vi "JSONHack.vi"(9 "search name":string, 11 "JSON in":string) -> (0 "Property (time stamp)":timestamp, 1 "Property (num)":dbl, 2 "Property (str)":string, 3 "What is left":string)   [LabVIEW 2019]
uses:
  <vilib>/Utility/miscctls.llb/LVDateTimeRec.ctl
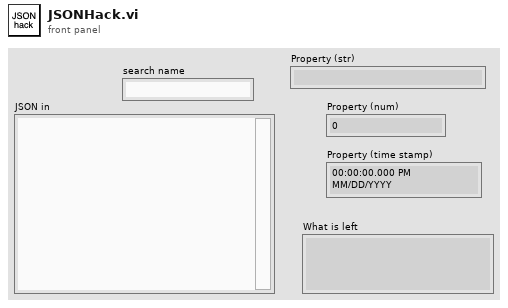
[diagram p1: front panel]
types:
  T1 = typedef "LVDateTimeRec.ctl" = cluster{"fractional second":dbl, "second":i32, "minute":i32, "hour":i32, "day of month":i32, "month":i32, "year":i32, "day of week":i32, "day of year":i32, "DST":i32}
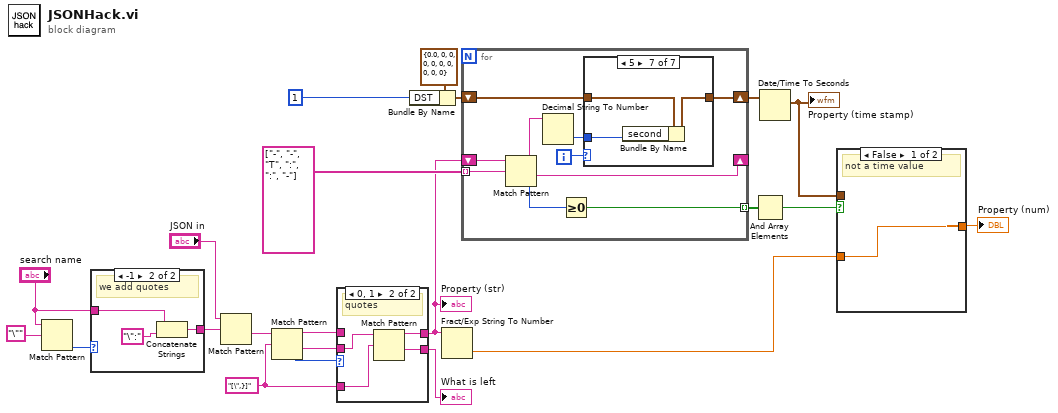
[diagram p0: block diagram]
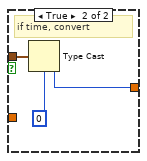
[diagram p2: hidden frame]
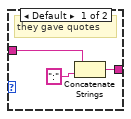
[diagram p4: hidden frame]
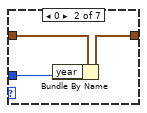
[diagram p6: hidden frame]
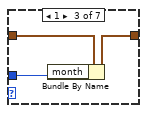
[diagram p7: hidden frame]
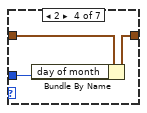
[diagram p8: hidden frame]
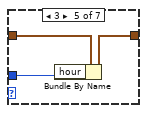
[diagram p9: hidden frame]
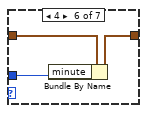
[diagram p10: hidden frame]
diagram:
  w9 = "[\",}]" ("regular expression")
  n1 = Match Pattern(string="search name", regular expression="\"" ("string")) -> (offset past match=w13:i32)  [unwired: 1 in, 3 out]
  n2 = case shown="-1" w13 {
    tunnel: [w24 w27] -> w20
    tunnel: "search name" -> [w23 w26]
    frame Default {
      # "they gave quotes"
      n3 = Concatenate Strings(w23, ":" ("string")) -> (w24:string)
    }
    frame -1 {
      # "we add quotes"
      n4 = Concatenate Strings(w26, "\":" ("string")) -> (w27:string)
    }
  }
  n5 = Match Pattern(string="JSON in", regular expression=w20) -> (after substring=w22:string)  [unwired: 1 in, 3 out]
  n6 = Match Pattern(string=w22, regular expression=w9) -> (before substring=w6:string, after substring=w10:string, offset past match=w11:i32)  [unwired: 1 in, 1 out]
  n7 = case shown="0, 1" w11 {
    tunnel: w10 -> [w30 w34]
    tunnel: w9 -> [_ w33]
    tunnel: [w30 w32] -> w8
    tunnel: [w29 w31] -> w7
    tunnel: w6 -> [w29 _]
    frame Default {
      # "number"
    }
    frame 0, 1 {
      # "quotes"
      n8 = Match Pattern(string=w34, regular expression=w33) -> (before substring=w31:string, after substring=w32:string)  [unwired: 1 in, 2 out]
    }
  }
  "Property (str)" <- w7
  "What is left" <- w8
  n9 = Bundle By Name(cluster=T1 {"fractional second"=0.0, "second"=0, "minute"=0, "hour"=0, "day of month"=0, "month"=0, "year"=0, "day of week"=0, "day of year"=0, "DST"=0} ("date time rec"), "DST"=1) -> (w15:T1)
  n10 = Fract/Exp String To Number(string=w7) -> (number=w3:dbl)  [unwired: 3 in, 1 out]
  n11 = for {
    tunnel: string[] ["-", "-", "T", ":", ":", "-"] -> [w43] mode=indexing
    shift-right: [w41] -> _
    shift-left: w7 -> [w44]
    shift-right: [w40] -> w18
    shift-left: w15 -> [w37]
    tunnel: [w35] -> w5 mode=indexing
    i -> [w39]
    n12 = Match Pattern(string=w44, regular expression=w43) -> (before substring=w42:string, after substring=w41:string, offset past match=w36:i32)  [unwired: 1 in, 1 out]
    n13 = Decimal String To Number(string=w42) -> (number=w38:i32)  [unwired: 2 in, 1 out]
    n14 = Greater Or Equal To 0?(x=w36) -> (x >= 0?=w35:bool)
    n15 = case shown="5" w39 {
      tunnel: w37 -> [w45 w48 w51 w54 w57 w60 w63]
      tunnel: [w45 w47 w50 w53 w56 w59 w62] -> w40
      tunnel: w38 -> [_ w46 w49 w52 w55 w58 w61]
      frame Default {
      }
      frame 0 {
        n16 = Bundle By Name(cluster=w48, "year"=w46) -> (w47:T1)
      }
      frame 1 {
        n17 = Bundle By Name(cluster=w51, "month"=w49) -> (w50:T1)
      }
      frame 2 {
        n18 = Bundle By Name(cluster=w54, "day of month"=w52) -> (w53:T1)
      }
      frame 3 {
        n19 = Bundle By Name(cluster=w57, "hour"=w55) -> (w56:T1)
      }
      frame 4 {
        n20 = Bundle By Name(cluster=w60, "minute"=w58) -> (w59:T1)
      }
      frame 5 {
        n21 = Bundle By Name(cluster=w63, "second"=w61) -> (w62:T1)
      }
    }
  }
  n22 = And Array Elements(Boolean array=w5) -> (logical AND=w4:bool)
  n23 = Date/Time To Seconds(2:w18) -> (0:w1:timestamp)  [unwired: 1 in]
  "Property (time stamp)" <- w1
  n24 = case shown="False" w4 {
    tunnel: w3 -> [w64 _]
    tunnel: [w64 w66] -> w2
    tunnel: w1 -> [_ w67]
    frame False {
      # "not a time value"
    }
    frame True {
      # "if time, convert"
      n25 = Type Cast(type=u64 0, x=w67) -> (*(type *) &x=w66:u64)
    }
  }
  "Property (num)" <- w2
